vi "Build Update Parameters.vi"(4 "TypeMap in":refnum<class "TypeMap.lvclass">, 8 "error in (no error)":errorcluster, 10 "object":variant, 11 "SqlMapper in":refnum<class "SqlMapper.lvclass">) -> (0 "error out":errorcluster, 1 "DynamicParameters out":refnum<class "DynamicParameters.lvclass">, 3 "SqlMapper out":refnum<class "SqlMapper.lvclass">)   [LabVIEW 2020, in "ORM.lvlib" / "TypeMap.lvclass"]
uses:
  TypeMap.lvclass
  DynamicParameters/DynamicParameters.lvclass
  SqlMapper/SqlMapper.lvclass
  TypeMap.lvclass/TypeMap.ctl
  DynamicParameters/DynamicParameters.lvclass/DynamicParameters.ctl
  DynamicParameters/Write KeyProperties.vi
  Read Autokey.vi
  Read KeyProperties.vi
  <vilib>/Utility/error.llb/Error Cluster From Error Code.vi
  <vilib>/ErrorRing/Error Ring.xnode
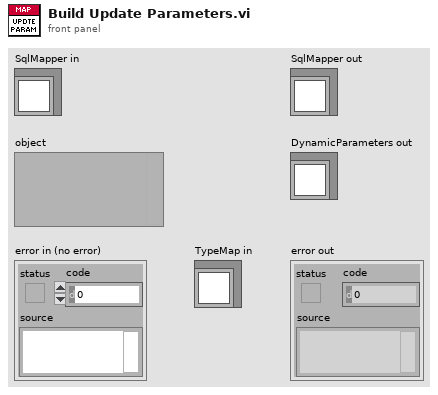
[diagram p1: front panel]
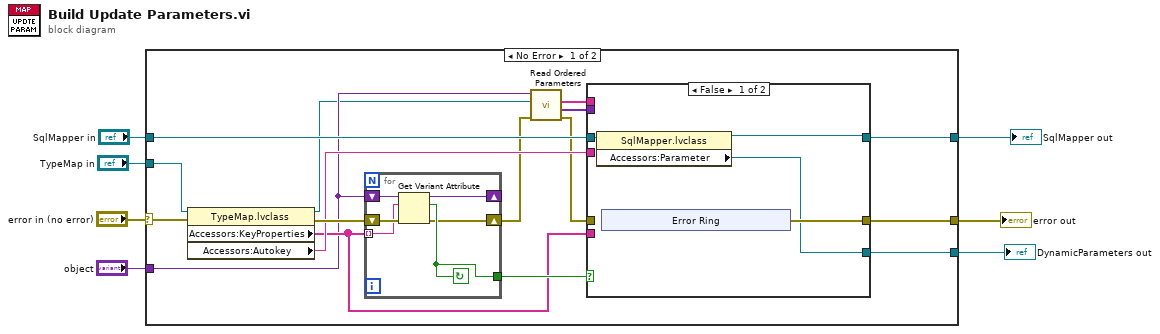
[diagram p0: block diagram]
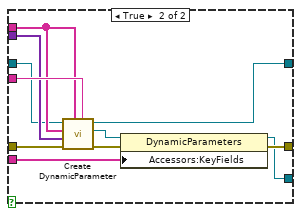
[diagram p2: hidden frame]
diagram:
  n1 = case shown="No Error" "error in (no error)" {
    selector: "error in (no error)" -> [w22 w50]
    tunnel: "TypeMap in" -> [w21 _]
    tunnel: "object" -> [w9 _]
    tunnel: "SqlMapper in" -> [w20 w51]
    tunnel: [w18 w51] -> w3
    tunnel: [w17 w50] -> w2
    tunnel: [w16 _] -> w1
    frame No Error {
      n2 = property class="TypeMap.lvclass"(reference=w21, error in=w22) -> (reference out=w8:refnum<class "TypeMap.lvclass">, error out=w23:errorcluster, "Accessors:KeyProperties"=w14:string[], "Accessors:Autokey"=w15:string)
      n3 = for {
        tunnel: w14 -> [w44] mode=indexing
        tunnel: [w48] -> w19
        shift-right: [w47] -> w13
        shift-left: w23 -> [w46]
        shift-right: [w45] -> _
        shift-left: w9 -> [w49]
        stop <- w48 continue-if-true
        n4 = Get Variant Attribute(Variant=w49, name=w44, error in=w46) -> (duplicate Variant=w45:variant, found=w48:bool, error out=w47:errorcluster)  [unwired: 1 in, 1 out]
      }
      n5 = call "Read Ordered Parameters.vi"("error in (no error)"=w13, "TypeMap in"=w8, "Object In"=w9) -> ("error out"=w12:errorcluster, "Values"=w11:variant[], "Fields"=w10:string[])  [unwired: 5 in, 1 out]
      n6 = case shown="False" w19 {
        tunnel: w12 -> [_ w43]
        tunnel: w20 -> [w26 w37]
        tunnel: [w25 w42] -> w18
        tunnel: [w27 w36] -> w17
        tunnel: [w24 w34] -> w16
        tunnel: w10 -> [_ w39]
        tunnel: w15 -> [_ w40]
        tunnel: w11 -> [_ w38]
        tunnel: w14 -> [_ w33]
        frame False {
          n7 = property class="SqlMapper.lvclass"(reference=w26) -> (reference out=w25:refnum<class "SqlMapper.lvclass">, "Accessors:Parameter"=w24:refnum<class "DynamicParameters.lvclass">)  [unwired: 1 in, 1 out]
          n8 = xnode "Error Ring"() -> ("error out"=w27:errorcluster)
        }
        frame True {
          n9 = call "Create DynamicParameter.vi"("AutoKey"=w40, "RequestedFields"=w39, "error in (no error)"=w43, "ParameterValues"=w38, "ParameterNames"=w39, "SqlMapper in"=w37) -> ("error out"=w41:errorcluster, "Parameters"=w35:refnum<class "DynamicParameters.lvclass">, "SqlMapper out"=w42:refnum<class "SqlMapper.lvclass">)  [unwired: 1 in, 2 out]
          n10 = property class="DynamicParameters"(reference=w35, error in=w41, "Accessors:KeyFields"=w33) -> (reference out=w34:refnum<class "DynamicParameters.lvclass">, error out=w36:errorcluster)
        }
      }
    }
    frame Error {
    }
  }
  "error out" <- w2
  "SqlMapper out" <- w3
  "DynamicParameters out" <- w1
